vi "Reset.vi"(8 "error in (no error)":errorcluster, 11 "TesteractHAL_DigitalIO In":refnum<class "TesteractHAL_DigitalOutput.lvclass">) -> (0 "error out":errorcluster, 3 "TesteractHAL_DigitalIO Out":refnum<class "TesteractHAL_DigitalOutput.lvclass">)   [LabVIEW 2017, in "TesteractHAL_DigitalOutput.lvlib" / "TesteractHAL_DigitalOutput.lvclass"]
doc: "Reset the device."
uses:
  TesteractHAL_DigitalOutput.lvclass
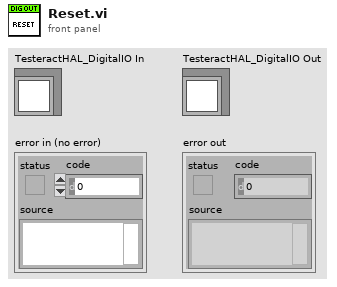
[diagram p1: front panel]
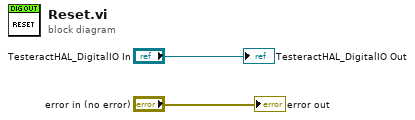
[diagram p0: block diagram]
diagram:
  "error out" <- "error in (no error)"
  "TesteractHAL_DigitalIO Out" <- "TesteractHAL_DigitalIO In"
